vi "_WCA_LO_REF_POW_OPT.vi"(6 "error in (no error)":errorcluster, 8 "LO_misc":T2={"LO FRQ(GHz)"=860.0, "LO multi "=9.0, "LocK?"=TRUE, "LO REF multi"=4.0, "wait (ms)"=100.0, "SG Pow Min (dBm)"=10.0, "SG Pow Max (dBm)"=20.0, "SG Pow Step (dBm)"=0.2, "SGPow OPT? "=TRUE, "SG set frq"=23.89638888888889, "SG set pow"=10.0}, 9 "Bias_LO_equip":T1={"Node address"=19, "CAN Interface"="CAN0", "Cartridge band"=10, "Slave Node in"={"Address"=0, "Serial Number"=[]}, "ObjHandle out"=0, "POL"=1, "sb"=1, "GPIB_SM (SIS S,V)"="24", "GPIB_DMM (SIS I)"="22", "GPIB_SM (MAG I) "="25", "GPIB_SG(LO)"="19", "GPIB_PW (PAMP) "="6", "GPIB_TMP1(8ch)"="12", "GPIB_TMP2(2ch)  "="13", "WCA_avg"=10, "Rsen"=10.0, "BiasModule"=1, "LOModule "=1, "WCA_LO_FREQ_SET"={"YTO Low freq. [GHz]"=14.42, "YTO High freq. [GHz]"=17.7, "Kvco"=1, "Lock Pol."=0, "SET LO FREQ"=72.5, "Multiplier"=6.0, "YTO (HEX)"=0, "YTO coarse( FREQ)"=25.0, "NULL PLL INTEGRATOR"=FALSE}, "Res for"=0} {"Res for" items=["none", "series res", "parallel res"]; "WCA_LO_FREQ_SET"."YTO coarse( FREQ)" min=25 max=150 step=0.0001 format="%.3f"; "WCA_LO_FREQ_SET"."Multiplier" min=3 max=6 step=3; "WCA_LO_FREQ_SET"."SET LO FREQ" min=25 max=150 step=0.0001 format="%.3f"; "WCA_LO_FREQ_SET"."Lock Pol." items=["Lower", "Upper"]; "WCA_LO_FREQ_SET"."Kvco" items=["7.5MHz/V", "15MHz/V"]; "WCA_LO_FREQ_SET"."YTO High freq. [GHz]" format="%.3f"; "WCA_LO_FREQ_SET"."YTO Low freq. [GHz]" format="%.3f"; "LOModule" items=["Manual", "B10Lab LO", "WCA LO"]; "BiasModule" items=["B10Lab Bias", "WCA BiasModule"]; "Slave Node in"."Serial Number" format="%.0x"; "Slave Node in"."Address" format="%.0x"; "Cartridge band" max=10 step=1; "Node address" format="%.0x"}) -> (0 "error out":errorcluster, 2 "LO_misc 2":T2={"LO FRQ(GHz)"=860.0, "LO multi "=9.0, "LocK?"=TRUE, "LO REF multi"=4.0, "wait (ms)"=100.0, "SG Pow Min (dBm)"=10.0, "SG Pow Max (dBm)"=20.0, "SG Pow Step (dBm)"=0.2, "SGPow OPT? "=TRUE, "SG set frq"=23.89638888888889, "SG set pow"=10.0})   [LabVIEW 2017]
panel:
  out "GET_PLL":T3={"PLL_ASSY_T"=34.469604, "PLL_REF_TOT_P"=-2.1142578, "PLL_IF_TOT_P"=-0.008850098, "PLL_CORR_V"=7.89376, "PLL_LOCK_V"=0.06496083, "PLL_5V_SUPPLY_V"=20.013428, "Temp_TF"=TRUE, "PLL Ref Pwr_TF"=TRUE, "IF Pwr_TF"=FALSE, "PLL Corr_TF"=FALSE, "PLL Lock V_TF"=FALSE, "PLL Nominal_TF"=FALSE}
  # "LO freq. [GHz]"
  # "YTO LOW\n/High Freq."
  # "ZERO Intgrtr"
  # "Node Address"
  # "Serial Number"
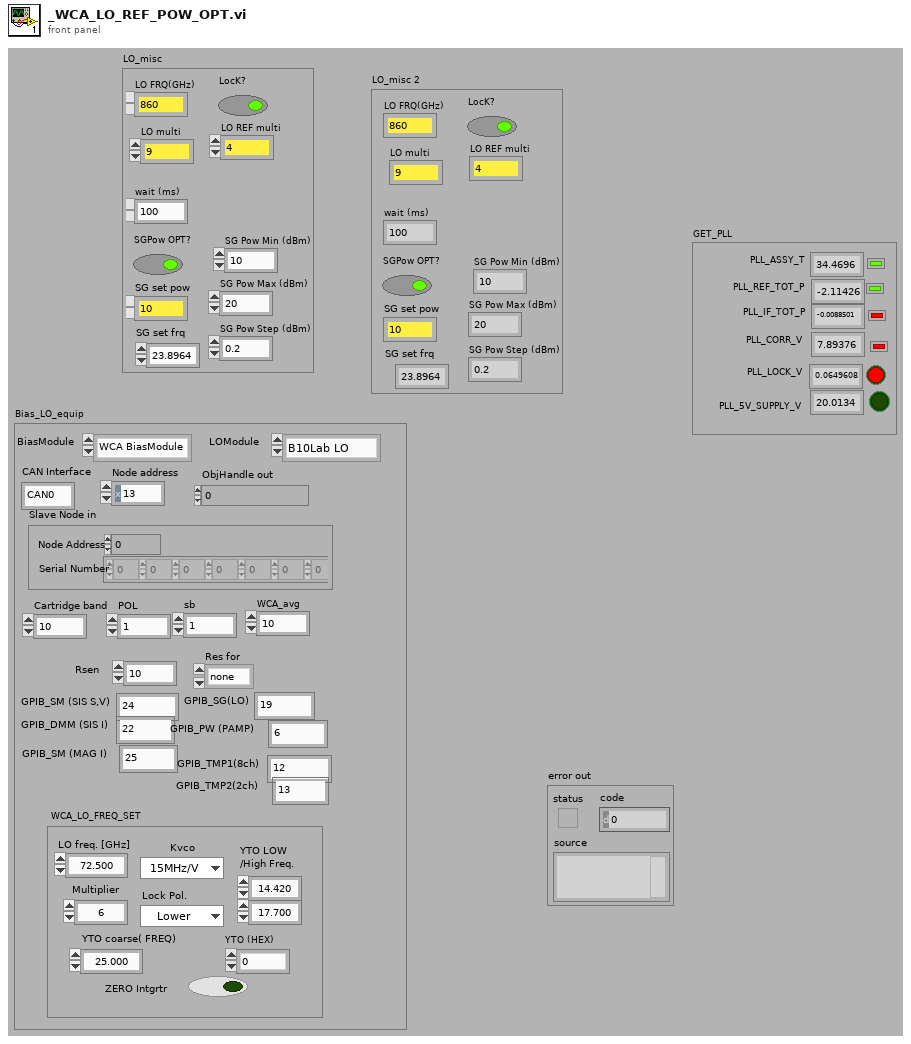
[diagram p1: front panel]
types:
  T1 = cluster{"Node address":u16, "CAN Interface":string, "Cartridge band":u32, "Slave Node in":cluster{"Address":i16, "Serial Number":i8[]}, "ObjHandle out":u32, "POL":u32, "sb":u32, "GPIB_SM (SIS S,V)":string, "GPIB_DMM (SIS I)":string, "GPIB_SM (MAG I) ":string, "GPIB_SG(LO)":string, "GPIB_PW (PAMP) ":string, "GPIB_TMP1(8ch)":string, "GPIB_TMP2(2ch)  ":string, "WCA_avg":i32, "Rsen":dbl, "BiasModule":u16, "LOModule ":u16, "WCA_LO_FREQ_SET":cluster{"YTO Low freq. [GHz]":sgl, "YTO High freq. [GHz]":sgl, "Kvco":u16, "Lock Pol.":u16, "SET LO FREQ":sgl, "Multiplier":sgl, "YTO (HEX)":u16, "YTO coarse( FREQ)":sgl, "NULL PLL INTEGRATOR":bool}, "Res for":u16}
  T2 = cluster{"LO FRQ(GHz)":dbl, "LO multi ":dbl, "LocK?":bool, "LO REF multi":dbl, "wait (ms)":dbl, "SG Pow Min (dBm)":dbl, "SG Pow Max (dBm)":dbl, "SG Pow Step (dBm)":dbl, "SGPow OPT? ":bool, "SG set frq":dbl, "SG set pow":dbl}
  T3 = cluster{"PLL_ASSY_T":sgl, "PLL_REF_TOT_P":sgl, "PLL_IF_TOT_P":sgl, "PLL_CORR_V":sgl, "PLL_LOCK_V":sgl, "PLL_5V_SUPPLY_V":sgl, "Temp_TF":bool, "PLL Ref Pwr_TF":bool, "IF Pwr_TF":bool, "PLL Corr_TF":bool, "PLL Lock V_TF":bool, "PLL Nominal_TF":bool}
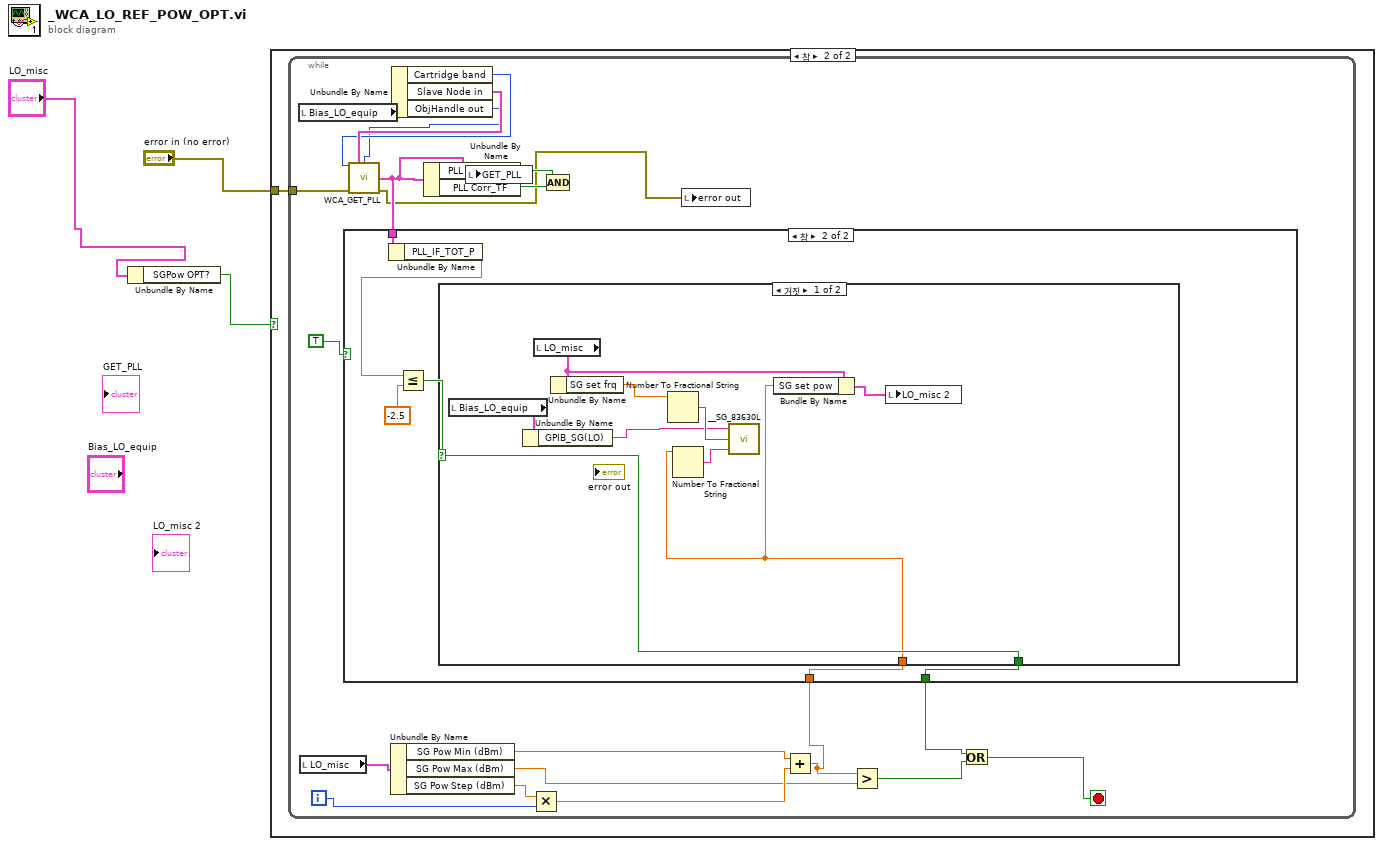
[diagram p0: block diagram]
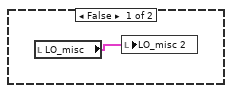
[diagram p2: hidden frame]
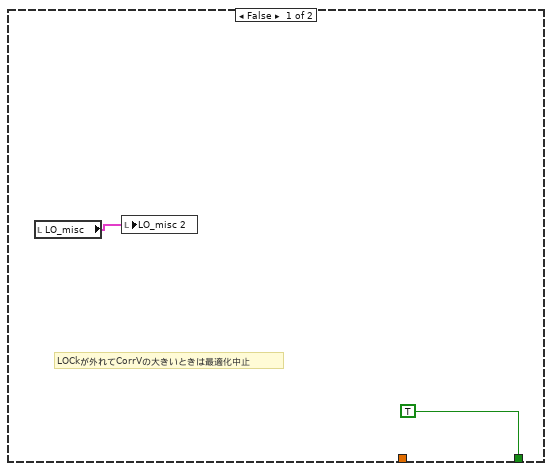
[diagram p3: hidden frame]
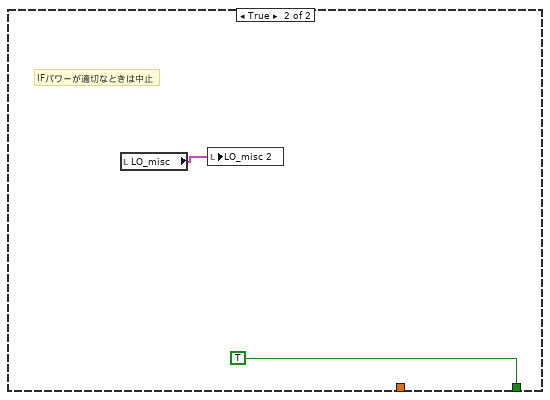
[diagram p4: hidden frame]
diagram:
  n1 = Unbundle By Name("LO_misc") -> ("SGPow OPT?"=w3:bool)
  n2 = case shown="참" w3 {
    tunnel: "error in (no error)" -> [_ w5]
    frame False {
      n3 = local read "LO_misc"() -> (w4:T2)
      n4 = local write "LO_misc 2"(w4) -> ()
    }
    frame True {
      n5 = while {
        tunnel: w5 -> [w15]
        i -> [w24]
        stop <- w19 stop-if-true
        n6 = local read "Bias_LO_equip"() -> (w14:T1)
        n7 = local read "LO_misc"() -> (w17:T2)
        n8 = Unbundle By Name(w17) -> ("SG Pow Min (dBm)"=w23:dbl, "SG Pow Max (dBm)"=w21:dbl, "SG Pow Step (dBm)"=w25:dbl)
        n9 = Unbundle By Name(w14) -> ("Cartridge band"=w12:u32, "Slave Node in"=w13:cluster{"Address":i16, "Serial Number":i8[]}, "ObjHandle out"=w11:u32)
        n10 = call "WCA_GET_PLL.vi"("Cartridge Band"=w12, "Slave Node in"=w13, "ObjHandle in"=w11, "error in (no error)"=w15) -> ("GET_PLL"=w8:T3, "error out"=w7:errorcluster)  [unwired: 9 in, 1 out]
        n11 = Unbundle By Name(w8) -> ("PLL Lock V_TF"=w10:bool, "PLL Corr_TF"=w9:bool)
        n12 = local write "GET_PLL"(w8) -> ()
        n13 = Multiply(x=w25, y=w24) -> (x*y=w22:dbl)
        n14 = Compound Arithmetic op=AND(w10, w9) -> ()  [unwired: 1 out]
        n15 = local write "error out"(w7) -> ()
        n16 = Add(x=w23, y=w22) -> (x+y=w16:dbl)
        n17 = case shown="참" TRUE {
          tunnel: [TRUE w33] -> w18
          tunnel: w8 -> [_ w32]
          tunnel: w16 -> [_ w31]
          frame False {
            # "LOCkが外れてCorrVの大きいときは最適化中止"
            n18 = local read "LO_misc"() -> (w26:T2)
            n19 = local write "LO_misc 2"(w26) -> ()
          }
          frame True {
            n20 = Unbundle By Name(w32) -> ("PLL_IF_TOT_P"=w30:sgl)
            n21 = Less Or Equal?(x=w30, y=-2.5) -> (x <= y?=w28:bool)
            n22 = case shown="거짓" w28 {
              selector: w28 -> [w39 _]
              tunnel: [w39 TRUE] -> w33
              tunnel: w31 -> [w36 _]
              frame False {
                n23 = local read "Bias_LO_equip"() -> (w35:T1)
                n24 = Unbundle By Name(w35) -> ("GPIB_SG(LO)"=w34:string)
                n25 = local read "LO_misc"() -> (w37:T2)
                n26 = Unbundle By Name(w37) -> ("SG set frq"=w40:dbl)
                n27 = Number To Fractional String(number=w40) -> (F-format string=w42:string)  [unwired: 3 in]
                n28 = Number To Fractional String(number=w36) -> (F-format string=w41:string)  [unwired: 3 in]
                n29 = call "__SG_83630L.vi"("PW(dBm)"=w41, "frq(GHz)"=w42, "GPIB"=w34) -> ()
                n30 = Bundle By Name(cluster=w37, "SG set pow"=w36) -> (w38:T2)
                n31 = local write "LO_misc 2"(w38) -> ()
              }
              frame True {
                # "IFパワーが適切なときは中止"
                n32 = local read "LO_misc"() -> (w43:T2)
                n33 = local write "LO_misc 2"(w43) -> ()
              }
            }
          }
        }
        n34 = Greater?(x=w16, y=w21) -> (0:w20:bool)
        n35 = Or(x=w18, y=w20) -> (x .or. y?=w19:bool)
      }
    }
  }
